vi "PH_uOPA_DelayController.panel.vi"(0 "object ref":refnum<vi>, 5 "error in (no error)":errorcluster) -> (19 "error out":errorcluster)   [LabVIEW 2014, in "PH_uOPA_DelayController.lvlib"]
doc: "This a GUI.\n\nLicense Agreement for this software:\n\nCopyright (C)\nGesellschaft für Schwerionenforschung, GSI\nPlanckstr. 1\n64291 Darmstadt\nGermany\n\nContact: D.Beck@gsi.de \n\nThis program is free software; you can redistribute it and/or modify it under the terms of the GNU General Public License as published by the Free Software Foundation; either version 2 of the license, or (at your option) any later version.\n\nThis program is distributed in the hope that it will be useful, but WITHOUT ANYW ARRANTY; without even the implied warranty of MERCHANTABILITY or FITNESS FOR A PARTICULAR PURPOSE. See the GNU General License for more details (http://www.gnu.org).\n\nGesellschaft für Schwerionenforschung, GSI\nPlanckstr. 1, 64291 Darmstadt, Germany\nFor all questions and ideas contact: M.Richter@gsi.de, H.Brand@gsi.de or D.Beck@gsi.de.\nLast update: 18-DEC-2002"
uses:
  PH_uOPA_DelayController.lvlib
  PH_Basics/PH_StatusHandler/PH_StatusHandler.GUI element.ctl
  PH_Devices/PH_TKTDS-30xx/PH_TKTDS-30xx.Channel Config.ctl
  PH_Devices/PH_TKTDS-30xx/PH_TKTDS-30xx.Waveform Limits.ctl
  PH_Devices/PH_TKTDS-30xx/PH_TKTDS-30xx.Acquisition Config.ctl
  PH_Devices/PH_TKTDS-30xx/PH_TKTDS-30xx.Trigger Config.ctl
  PH_Basics/PH_Stepmotor_BaseClass/PH_Stepmotor_BaseClass.Axis Settings.ctl
  PH_Basics/PH_Stepmotor_BaseClass/PH_Stepmotor_BaseClass.Motor Type.ctl
  PH_Basics/PH_Stepmotor_BaseClass/PH_Stepmotor_BaseClass.Axis Address.ctl
  PH_Basics/PH_Stepmotor_BaseClass/PH_Stepmotor_BaseClass.Axis Activity.ctl
  PH_uOPA_DelayController.Limit.ctl
  PH_uOPA_DelayController.Control Status.ctl
  PH_Devices/PH_TKTDS-30xx/PH_TKTDS-30xx.GUI Refs.ctl
  PH_Basics/PH_AxisGUI_BaseClass/PH_AxisGUI_BaseClass.Axis GUI Refs.ctl
  PH_Basics/PH_Stepmotor_BaseClass/PH_Stepmotor_BaseClass.Axis Direction.ctl
  CS_Core/CSObj/CSObj.lvlib
  PH_Basics/PH_Common/PH_Common.lvlib
  CS_Core/CSSystem/CSSystemLib/CSSystemLib.lvlib
  PH_Devices/PH_TKTDS-30xx/PH_TKTDS-30xx.lvlib
  PH_Basics/PH_Class/PH_Class.lvlib
  PH_Basics/PH_StatusHandler/PH_StatusHandler.lvlib
  PH_Basics/PH_AxisGUI_BaseClass/PH_AxisGUI_BaseClass.lvlib
  PH_Basics/PH_Stepmotor_BaseClass/PH_Stepmotor_BaseClass.lvlib
panel:
  in  "Stop":bool caption="SetZero"
  out "VISA Resource":string
  out "State":u32(colorbox)
  in  "Tab Control":T1(tab)
  out "Current uOPA Mean":dbl caption="uOPA Mean"
  out "Control Status":T2
  in  "Control":bool
  out "Pump running":bool
  in  "Pump Limit [%]":dbl caption="Limit [%]"
  in  "Pump Target":dbl caption="Target"
  in  "uOPA Target":dbl caption="Target"
  in  "uOPA Limits [%]":T3 caption="Limits [%]"
  out "Current uOPA Peak":dbl caption="uOPA Peak"
  out "Current Pump Peak":dbl caption="Pump Peak" format="%_4f"
  out "Activity":T4
  out "Motion Status Bar":u32(colorbox)=16777088 caption="Axis1"
  out "Motion Status":u32(colorbox)=6618880 caption="Axis1"
  in  "Clear Error":bool
  in  "Forth":bool caption="? Steps"
  in  "Back":bool caption="? Steps"
  in  "Target":string="0" caption="Steps"
  out "Trace Pump":waveform(dbl)[](graph)
  out "Trace uOPA":waveform(dbl)[](graph)
  in  "Samples":i32=100
  out "uOPA Mean":dbl(graph)
  out "Pump Peak":dbl(graph)
  out "uOPA Peak":dbl(graph)
  out "Address":T5={"Instance"="N/A", "Motor Nr"=0}
  in  "SetZero":bool
  in  "Reset":bool
  in  "Settings":T6={"Sign change"=FALSE, "Width"=0.0, "Calibration"=0.0, "Unit"="Steps", "Motor Type"=enum."Unspecific", "Unit Width"="", "Unit CF"=""}
  in  "Trigger":T8={"Source"="CH1", "Slope"=0, "Level [V]"=0.0} {"Level [V]" format="%#_6p"}
  in  "Acquisition":T9={"Time base"=2e-07, "Record Length"=10000, "Start Time"=0.0, "Type"=0, "Continuous"=FALSE} {"Start Time" format="%#_12p"; "Record Length" items=["500"=500, "10000"=10000]; "Time base" items=["2ns"=2e-09, "4ns"=4e-09, "10ns"=1e-08, "20ns"=2e-08, "40ns"=4e-08, "100ns"=1e-07, "200ns"=2e-07, "400ns"=4e-07, "1µs"=1e-06, "2µs"=2e-06, "4µs"=4e-06, "10µs"=1e-05, "20µs"=2e-05, "40µs"=4e-05, "100µs"=0.0001, "200µs"=0.0002, "400µs"=0.0004, "1ms"=0.001, "2ms"=0.002, "10ms"=0.01, "20ms"=0.02, "40ms"=0.04, "100ms"=0.1, "200ms"=0.2, "400ms"=0.4, "1s"=1.0, "2s"=2.0, "4s"=4.0, "10s"=10.0]}
  in  "Pump":T10={"Channel Name"="CH1", "Input Impedance"="MEG", "Max Input Frequency"="TWENTY", "Vertical Coupling"=1, "Channel Enabled"=TRUE, "Probe Attenuation"=1.0, "Vertical Range"=100.0, "Vertical Offset"=0.0, "Waveform Limits"={"Start"=1, "End"=10000}} {"Vertical Offset" format="%#_6p"; "Vertical Range" items=["1mV"=0.001, "2mV"=0.002, "5mV"=0.005, "10mV"=0.01, "20mV"=0.02, "50mV"=0.05, "100mV"=0.1, "200mV"=0.2, "500mV"=0.5, "1V"=1.0]; "Probe Attenuation" format="%#.2f"}
  in  "uOPA":T10={"Channel Name"="CH1", "Input Impedance"="MEG", "Max Input Frequency"="TWENTY", "Vertical Coupling"=1, "Channel Enabled"=TRUE, "Probe Attenuation"=1.0, "Vertical Range"=100.0, "Vertical Offset"=0.0, "Waveform Limits"={"Start"=1, "End"=10000}} {"Vertical Offset" format="%#_6p"; "Vertical Range" items=["1mV"=0.001, "2mV"=0.002, "5mV"=0.005, "10mV"=0.01, "20mV"=0.02, "50mV"=0.05, "100mV"=0.1, "200mV"=0.2, "500mV"=0.5, "1V"=1.0]; "Probe Attenuation" format="%#.2f"}
  in  "Position":dbl
  in  "Channel to be positioned":string(combo)="CH1"
  in  "Display Intensity":u8=1 min=1 max=100 step=1
  out "PSDB Status":u32(colorbox)=6618880 caption="PSDB"
  out "Status":T12 caption="Enabling State"
  in  "Delete":bool
  in  "Exit":bool
  # "PCS"
  # "3.40"
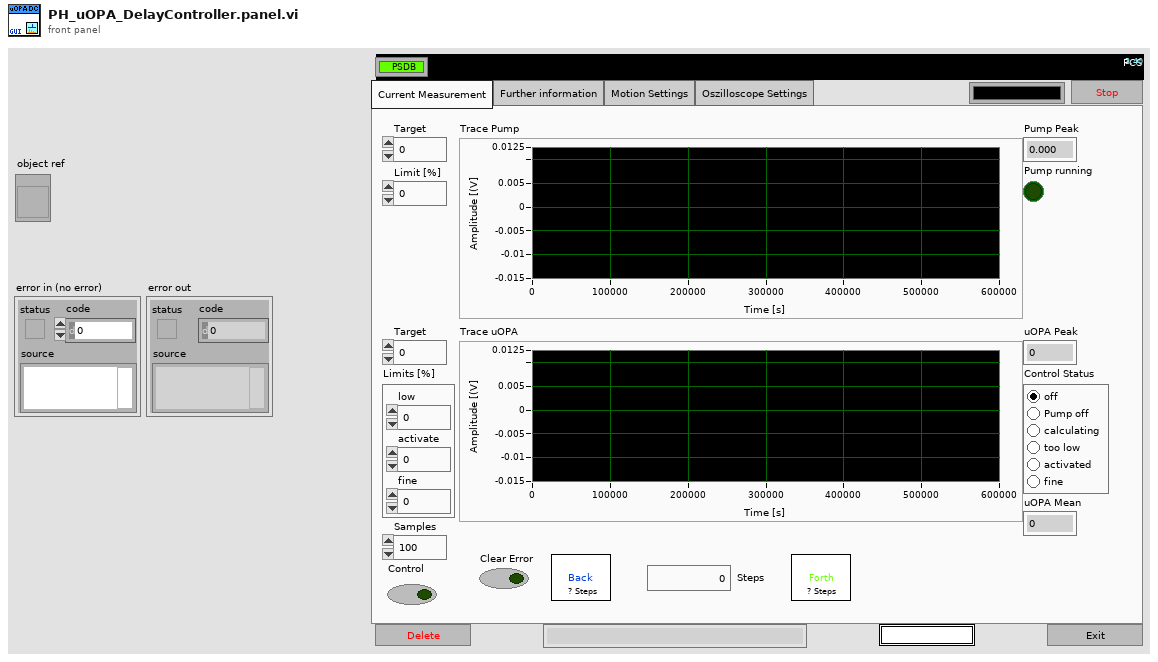
[diagram p1: front panel]
types:
  T1 = enum32{"Current Measurement", "Further information", "Motion Settings", "Oszilloscope Settings"}
  T2 = typedef "PH_uOPA_DelayController.lvlib/PH_uOPA_DelayController.Control Status.ctl" = enum32{"off", "Pump off", "calculating", "too low", "activated", "fine"}
  T3 = typedef "PH_uOPA_DelayController.lvlib/PH_uOPA_DelayController.Limit.ctl" = cluster{"low":dbl, "activate":dbl, "fine":dbl}
  T4 = typedef "PH_Stepmotor_BaseClass.lvlib/PH_Stepmotor_BaseClass.Axis Activity.ctl" = enum16{"No Information", "stopped", "running", "Failure", "Alarm", "stopped at backward ES", "stopped at foreward ES"}
  T5 = typedef "PH_Stepmotor_BaseClass.lvlib/PH_Stepmotor_BaseClass.Axis Address.ctl" = cluster{"Instance":string, "Motor Nr":i32}
  T6 = typedef "PH_Stepmotor_BaseClass.lvlib/PH_Stepmotor_BaseClass.Axis Settings.ctl" = cluster{"Sign change":bool, "Width":dbl, "Calibration":dbl, "Unit":string, "Motor Type":T7, "Unit Width":string, "Unit CF":string}
  T7 = typedef "PH_Stepmotor_BaseClass.lvlib/PH_Stepmotor_BaseClass.Motor Type.ctl" = enum16{"Unspecific", "OWIS 49.120.2633", "OWIS 49.060.1033", "OWIS 43.040.2558", "Diamond Motion 2200 series", "OWIS 49.120.266B.MV6", "Calorimeter", "Linear Stage 1", "MICOS VT-80", "MICOS VT-80 S", "Standa Rotstage nt0.95A", "PUF RA 320.200", "PUF RA 800.200", "PUF RA 800.400", "PUF RA 400.50", "1324.nn.800.50", "1324.n9c.800.50", "1324.nn.320.200", "1324.nn.400.200", "1324.nn.800.200", "1324.nn.400.50", "1324.8c9c.800.50", "1324.8c9c.400.200"}
  T8 = typedef "PH_TKTDS-30xx.lvlib/PH_TKTDS-30xx.Trigger Config.ctl" = cluster{"Source":string, "Slope":i32, "Level [V]":dbl}
  T9 = typedef "PH_TKTDS-30xx.lvlib/PH_TKTDS-30xx.Acquisition Config.ctl" = cluster{"Time base":dbl, "Record Length":u16, "Start Time":dbl, "Type":i32, "Continuous":bool}
  T10 = typedef "PH_TKTDS-30xx.lvlib/PH_TKTDS-30xx.Channel Config.ctl" = cluster{"Channel Name":string, "Input Impedance":string, "Max Input Frequency":string, "Vertical Coupling":i32, "Channel Enabled":bool, "Probe Attenuation":dbl, "Vertical Range":dbl, "Vertical Offset":dbl, "Waveform Limits":T11}
  T11 = typedef "PH_TKTDS-30xx.lvlib/PH_TKTDS-30xx.Waveform Limits.ctl" = cluster{"Start":i32, "End":i32}
  T12 = typedef "PH_StatusHandler.lvlib/PH_StatusHandler.GUI element.ctl" = u16
  T13 = typedef "PH_AxisGUI_BaseClass.lvlib/PH_AxisGUI_BaseClass.Axis GUI Refs.ctl" = cluster{"Back":refnum<vi>, "Forth":refnum<vi>, "Status":refnum<vi>, "Target":refnum<vi>, "Address":refnum<vi>, "Status Bar":refnum<vi>, "Settings":refnum<vi>, "Activity":refnum<vi>, "Clear Error":refnum<vi>}
  T14 = typedef "PH_TKTDS-30xx.lvlib/PH_TKTDS-30xx.GUI Refs.ctl" = cluster{"Trigger":refnum<vi>, "Acquisition":refnum<vi>, "State":refnum<vi>, "Delete":refnum<vi>, "Channel to be positioned":refnum<vi>, "Postion":refnum<vi>, "Display Intensity":refnum<vi>, "VISA Resource":refnum<vi>, "Channels":refnum<vi>[], "Graphs":refnum<vi>[]}
  T15 = typedef "PH_Stepmotor_BaseClass.lvlib/PH_Stepmotor_BaseClass.Axis Direction.ctl" = enum16{"forward", "backward"}
  T16 = typedef "PH_AxisGUI_BaseClass.lvlib/PH_AxisGUI_BaseClass.i attribute.ctl" = cluster{"Axes":T17[]}
  T17 = typedef "PH_AxisGUI_BaseClass.lvlib/PH_AxisGUI_BaseClass.Axis Attributes.ctl" = cluster{"Axis GUI Refs":T13, "Address":T5, "Name":string, "Label \"Back\"":string, "Labell \"Forth\"":string, "Moving?":bool}
  T18 = typedef "PH_uOPA_DelayController.lvlib/PH_uOPA_DelayController.i attribute.ctl" = cluster{"GUI Refs":cluster{"Current Pump Peak":refnum<vi>, "Current uOPA Peak":refnum<vi>, "Pump Peak":refnum<vi>, "uOPA Peak":refnum<vi>, "uOPA Target":refnum<vi>, "uOPA Limits [%]":refnum<vi>, "sample length":refnum<vi>, "Pump Target":refnum<vi>, "Pump Limit":refnum<vi>, "Pump running":refnum<vi>, "Feedback Control":refnum<vi>, "Control Status":refnum<vi>, "uOPA Mean":refnum<vi>, "Current uOPA Mean":refnum<vi>}, "uOPA Target":dbl, "uOPA Limits [%]":T3, "Sample Length":i32, "Initialize Mean":bool, "Pump Target":dbl, "Pump Limit [%]":dbl, "Feedback Control":bool, "Control Status":T2, "last Mean":dbl, "last direction":T15, "Axis Settings":T6, "Width while feedback":dbl}
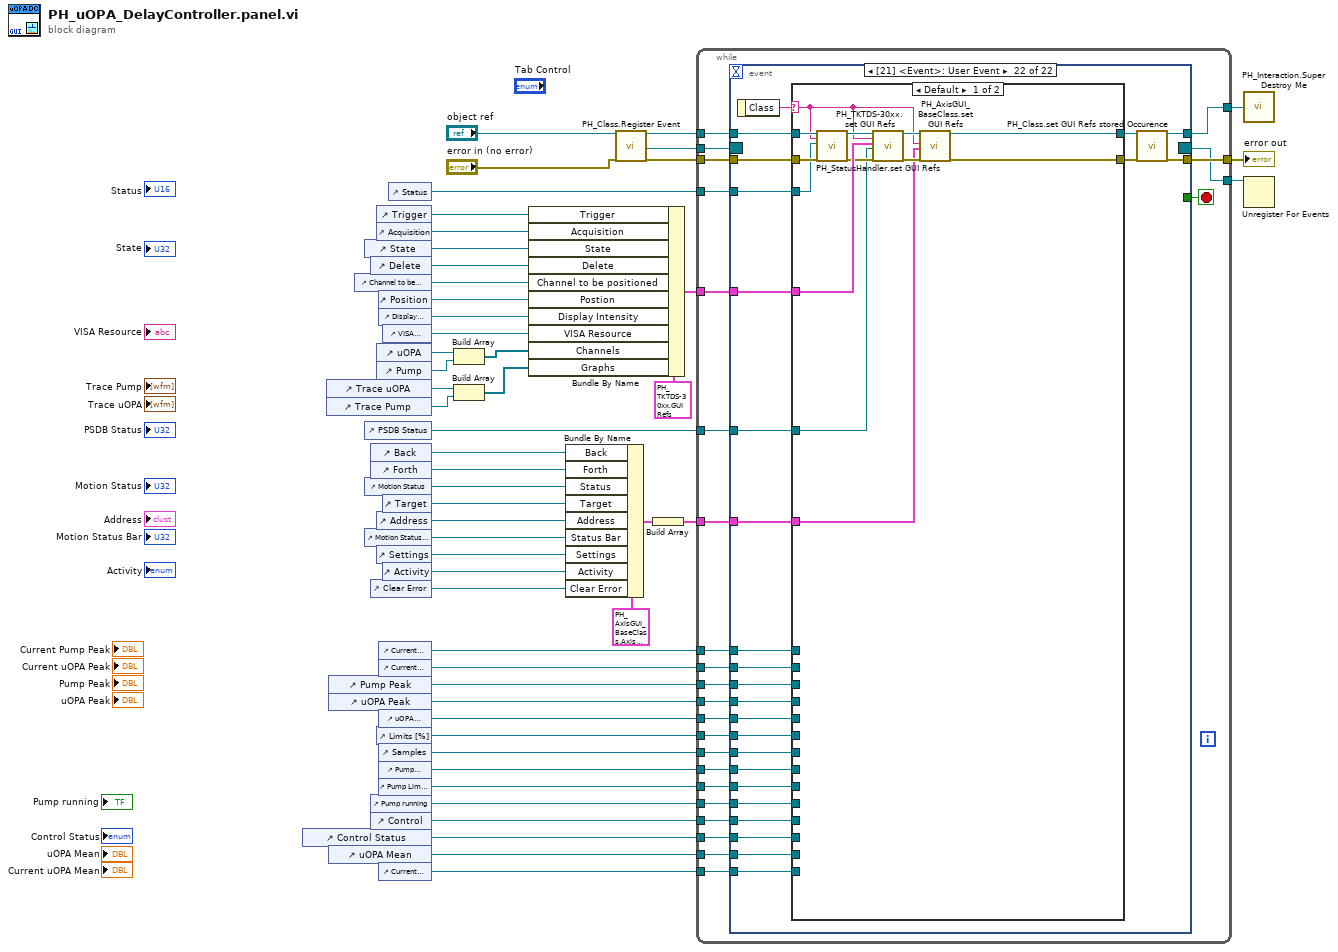
[diagram p0: block diagram]
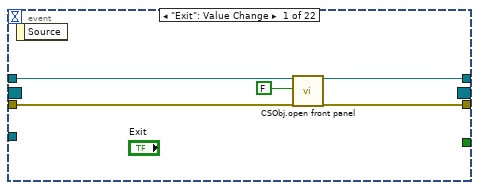
[diagram p2: hidden frame]
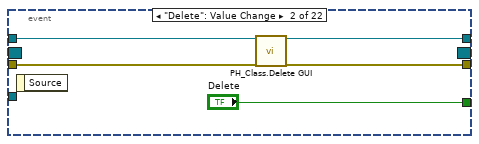
[diagram p3: hidden frame]
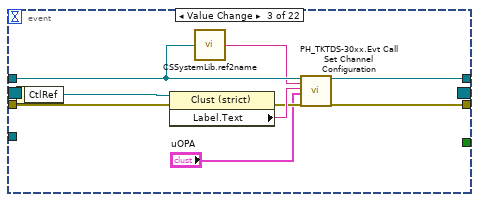
[diagram p4: hidden frame]
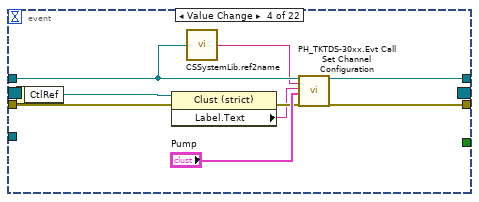
[diagram p5: hidden frame]
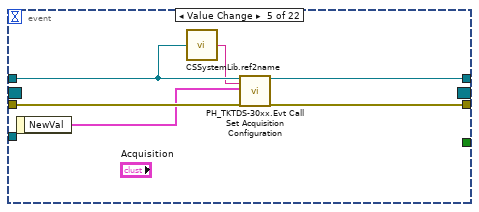
[diagram p6: hidden frame]
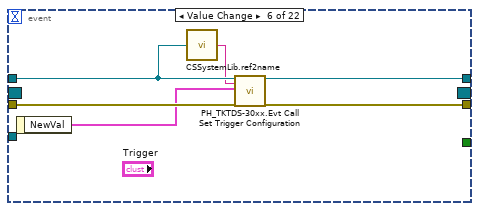
[diagram p7: hidden frame]
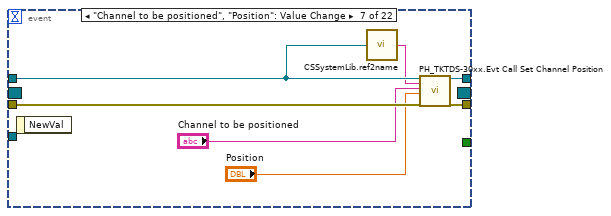
[diagram p8: hidden frame]
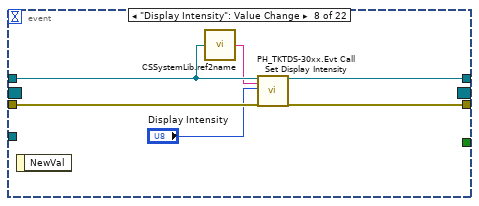
[diagram p9: hidden frame]
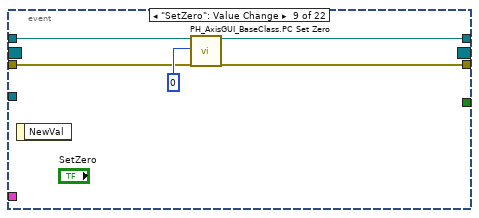
[diagram p10: hidden frame]
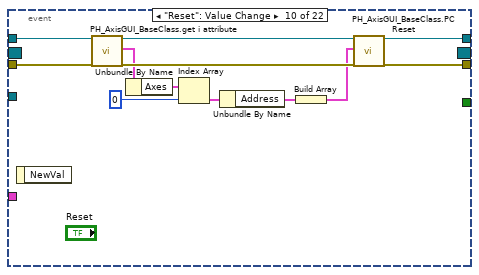
[diagram p11: hidden frame]
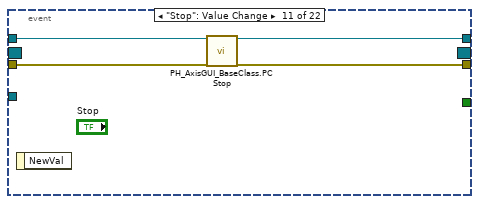
[diagram p12: hidden frame]
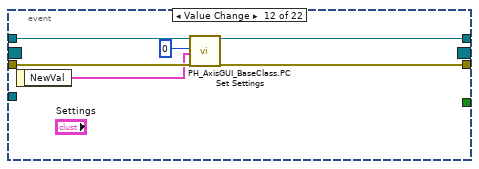
[diagram p13: hidden frame]
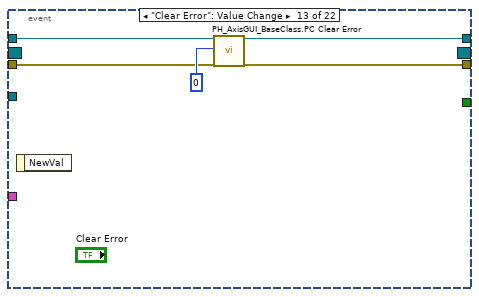
[diagram p14: hidden frame]
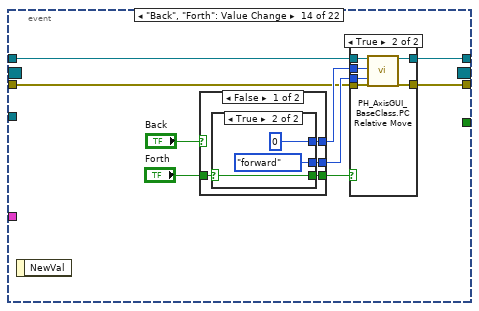
[diagram p15: hidden frame]
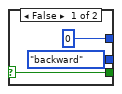
[diagram p16: hidden frame]
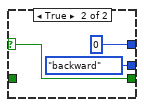
[diagram p17: hidden frame]
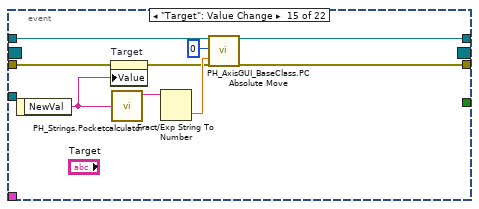
[diagram p19: hidden frame]
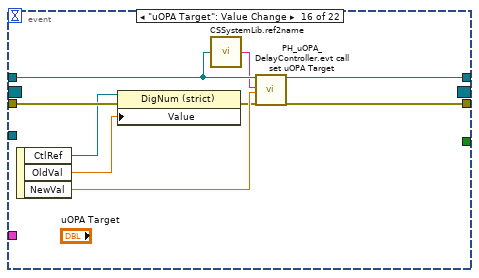
[diagram p20: hidden frame]
diagram:
  n1 = control-ref of="Control Status"() -> (w3:refnum<vi>)
  n2 = control-ref of="Trace uOPA"() -> (w17:refnum<vi>)
  n3 = control-ref of="Trace Pump"() -> (w16:refnum<vi>)
  n4 = control-ref of="Pump Peak"() -> (w12:refnum<vi>)
  n5 = control-ref of="uOPA Peak"() -> (w11:refnum<vi>)
  n6 = control-ref of="uOPA Mean"() -> (w2:refnum<vi>)
  n7 = control-ref of="Channel to be positioned"() -> (w43:refnum<vi>)
  n8 = control-ref of="State"() -> (w45:refnum<vi>)
  n9 = control-ref of="PSDB Status"() -> (w18:refnum<vi>)
  n10 = control-ref of="Motion Status"() -> (w26:refnum<vi>)
  n11 = control-ref of="Motion Status Bar"() -> (w27:refnum<vi>)
  n12 = control-ref of="Delete"() -> (w48:refnum<vi>)
  n13 = control-ref of="Back"() -> (w21:refnum<vi>)
  n14 = control-ref of="Forth"() -> (w20:refnum<vi>)
  n15 = control-ref of="Clear Error"() -> (w19:refnum<vi>)
  n16 = control-ref of="Pump running"() -> (w5:refnum<vi>)
  n17 = control-ref of="Control"() -> (w4:refnum<vi>)
  n18 = control-ref of="Trigger"() -> (w47:refnum<vi>)
  n19 = control-ref of="Acquisition"() -> (w46:refnum<vi>)
  n20 = control-ref of="uOPA"() -> (w50:refnum<vi>)
  n21 = control-ref of="Pump"() -> (w49:refnum<vi>)
  n22 = control-ref of="Address"() -> (w24:refnum<vi>)
  n23 = control-ref of="Settings"() -> (w23:refnum<vi>)
  n24 = control-ref of="Limits [%]"() -> (w9:refnum<vi>)
  n25 = control-ref of="Position"() -> (w42:refnum<vi>)
  n26 = control-ref of="Display Intensity"() -> (w44:refnum<vi>)
  n27 = control-ref of="Current Pump Peak"() -> (w14:refnum<vi>)
  n28 = control-ref of="Current uOPA Peak"() -> (w13:refnum<vi>)
  n29 = control-ref of="uOPA Target"() -> (w10:refnum<vi>)
  n30 = control-ref of="Samples"() -> (w8:refnum<vi>)
  n31 = control-ref of="Pump Target"() -> (w7:refnum<vi>)
  n32 = control-ref of="Pump Limit [%]"() -> (w6:refnum<vi>)
  n33 = control-ref of="Current uOPA Mean"() -> (w1:refnum<vi>)
  n34 = control-ref of="VISA Resource"() -> (w41:refnum<vi>)
  n35 = control-ref of="Target"() -> (w22:refnum<vi>)
  n36 = control-ref of="Activity"() -> (w25:refnum<vi>)
  n37 = control-ref of="Status"() -> (w31:refnum<vi>)
  n38 = Build Array(w50, w49) -> (w35:refnum<vi>[])
  n39 = Build Array(w17, w16) -> (w15:refnum<vi>[])
  n40 = Bundle By Name(cluster=T14 {"Trigger"=refnum, "Acquisition"=refnum, "State"=refnum, "Delete"=refnum, "Channel to be positioned"=refnum, "Postion"=refnum, "Display Intensity"=refnum, "VISA Resource"=refnum, "Channels"=[], "Graphs"=[]} ("GUI Refs"), "Trigger"=w47, "Acquisition"=w46, "State"=w45, "Delete"=w48, "Channel to be positioned"=w43, "Postion"=w42, "Display Intensity"=w44, "VISA Resource"=w41, "Channels"=w35, "Graphs"=w15) -> (w34:T14)
  n41 = Bundle By Name(cluster=T13 {"Back"=refnum, "Forth"=refnum, "Status"=refnum, "Target"=refnum, "Address"=refnum, "Status Bar"=refnum, "Settings"=refnum, "Activity"=refnum, "Clear Error"=refnum} ("GUI Refs"), "Back"=w21, "Forth"=w20, "Status"=w26, "Target"=w22, "Address"=w24, "Status Bar"=w27, "Settings"=w23, "Activity"=w25, "Clear Error"=w19) -> (w29:T13)
  n42 = call "PH_Class.Register Event.vi"("i ref in"="object ref", "error in (no error)"="error in (no error)") -> ("i ref out"=w40:refnum<vi>, "Event Registration Refnum"=w38:refnum<event-registration>, "error out"=w39:errorcluster)  [unwired: 15 in]
  n43 = Build Array(w29) -> (w28:T13[])
  n44 = while {
    tunnel: w40 -> [w74]
    tunnel: [w73] -> w52
    tunnel: w39 -> [w76]
    tunnel: [w75] -> w51
    tunnel: w38 -> [w72]
    tunnel: [w71] -> w37
    tunnel: w31 -> [w70]
    tunnel: w34 -> [w69]
    tunnel: w28 -> [w68]
    tunnel: w18 -> [w67]
    tunnel: w14 -> [w66]
    tunnel: w13 -> [w65]
    tunnel: w12 -> [w64]
    tunnel: w11 -> [w63]
    tunnel: w10 -> [w62]
    tunnel: w9 -> [w61]
    tunnel: w8 -> [w60]
    tunnel: w7 -> [w59]
    tunnel: w6 -> [w58]
    tunnel: w5 -> [w57]
    tunnel: w4 -> [w56]
    tunnel: w3 -> [w55]
    tunnel: w2 -> [w54]
    tunnel: w1 -> [w53]
    stop <- w77 stop-if-true
    n45 = event shown="[21] <Event>: User Event" {
      selector: w72 -> [_ _ _ _ _ _ _ _ _ _ _ _ _ _ _ _ _ _ _ _ _ _]
      dyn-events: [_ _ _ _ _ _ _ _ _ _ _ _ _ _ _ _ _ _ _ _ _ _] -> w71
      timeout: _ -> [_ _ _ _ _ _ _ _ _ _ _ _ _ _ _ _ _ _ _ _ _ _]
      tunnel: [_ "Delete" _ _ _ _ _ _ _ _ _ _ _ _ _ _ _ _ _ _ _ _] -> w77
      tunnel: w74 -> [w79 w84 w94 w103 w108 w114 w121 w127 w134 w139 w151 w156 w161 w168 w198 w207 w216 w225 w234 w243 w252 w278]
      tunnel: w76 -> [w82 w86 w90 w98 w111 w117 w124 w130 w133 w137 w150 w154 w160 w166 w197 w210 w219 w228 w237 w246 w255 w277]
      tunnel: [w81 w85 w96 w105 w110 w116 w123 w129 w131 w136 w148 w153 w158 w165 w194 w208 w217 w226 w235 w244 w253 w279] -> w75
      tunnel: [w78 w83 w95 w104 w109 w115 w122 w128 w132 w138 w149 w155 w159 w167 w195 w209 w218 w227 w236 w245 w254 w280] -> w73
      tunnel: w70 -> [_ _ _ _ _ _ _ _ _ _ _ _ _ _ _ _ _ _ _ _ _ w274]
      tunnel: w69 -> [_ _ _ _ _ _ _ _ _ _ _ _ _ _ _ _ _ _ _ _ _ w272]
      tunnel: w68 -> [_ _ _ _ _ _ _ _ _ _ _ _ _ _ _ _ _ _ _ _ _ w271]
      tunnel: w67 -> [_ _ _ _ _ _ _ _ _ _ _ _ _ _ _ _ _ _ _ _ _ w270]
      tunnel: w66 -> [_ _ _ _ _ _ _ _ _ _ _ _ _ _ _ _ _ _ _ _ _ w269]
      tunnel: w65 -> [_ _ _ _ _ _ _ _ _ _ _ _ _ _ _ _ _ _ _ _ _ w268]
      tunnel: w64 -> [_ _ _ _ _ _ _ _ _ _ _ _ _ _ _ _ _ _ _ _ _ w267]
      tunnel: w63 -> [_ _ _ _ _ _ _ _ _ _ _ _ _ _ _ _ _ _ _ _ _ w266]
      tunnel: w62 -> [_ _ _ _ _ _ _ _ _ _ _ _ _ _ _ _ _ _ _ _ _ w265]
      tunnel: w61 -> [_ _ _ _ _ _ _ _ _ _ _ _ _ _ _ _ _ _ _ _ _ w264]
      tunnel: w60 -> [_ _ _ _ _ _ _ _ _ _ _ _ _ _ _ _ _ _ _ _ _ w263]
      tunnel: w59 -> [_ _ _ _ _ _ _ _ _ _ _ _ _ _ _ _ _ _ _ _ _ w262]
      tunnel: w58 -> [_ _ _ _ _ _ _ _ _ _ _ _ _ _ _ _ _ _ _ _ _ w261]
      tunnel: w57 -> [_ _ _ _ _ _ _ _ _ _ _ _ _ _ _ _ _ _ _ _ _ w260]
      tunnel: w56 -> [_ _ _ _ _ _ _ _ _ _ _ _ _ _ _ _ _ _ _ _ _ w259]
      tunnel: w55 -> [_ _ _ _ _ _ _ _ _ _ _ _ _ _ _ _ _ _ _ _ _ w258]
      tunnel: w54 -> [_ _ _ _ _ _ _ _ _ _ _ _ _ _ _ _ _ _ _ _ _ w257]
      tunnel: w53 -> [_ _ _ _ _ _ _ _ _ _ _ _ _ _ _ _ _ _ _ _ _ w256]
      event "Exit": Value Change {
        n46 = event-data() -> ()  [unwired: 1 in, 1 out]
        n47 = call "CSObj.open front panel.vi"("i ref in"=w79, "frontPanelOpen"=FALSE ("front panel open"), "error in (no error)"=w82) -> ("i ref out"=w78:refnum<vi>, "error out"=w81:errorcluster)  [unwired: 15 in]
      }
      event "Delete": Value Change {
        n48 = event-data() -> ()  [unwired: 1 in, 1 out]
        n49 = call "PH_Class.Delete GUI.vi"("VI in"=w84, "error in (no error)"=w86) -> ("VI out"=w83:refnum<vi>, "error out"=w85:errorcluster)  [unwired: 16 in]
      }
      event Value Change {
        n50 = event-data() -> ("CtlRef"=w93:refnum<vi>)  [unwired: 1 in]
        n51 = property class="Clust (strict)"(reference=w93, error in=w90) -> (error out=w89:errorcluster, "Label.Text"=w91:string)  [unwired: 1 out]
        n52 = call "CSSystemLib.ref2name.vi"("obj refnum"=w94) -> ("name"=w92:string)
        n53 = call "PH_TKTDS-30xx.Evt Call Set Channel Configuration.vi"("i ref in"=w94, "Instance"=w92, "GUI Element Name"=w91, "Channel Configuration"="uOPA", "error in (no error)"=w89) -> ("i ref out"=w95:refnum<vi>, "error out"=w96:errorcluster)  [unwired: 13 in]
      }
      event Value Change {
        n54 = event-data() -> ("CtlRef"=w100:refnum<vi>)  [unwired: 1 in]
        n55 = property class="Clust (strict)"(reference=w100, error in=w98) -> (error out=w99:errorcluster, "Label.Text"=w97:string)  [unwired: 1 out]
        n56 = call "CSSystemLib.ref2name.vi"("obj refnum"=w103) -> ("name"=w102:string)
        n57 = call "PH_TKTDS-30xx.Evt Call Set Channel Configuration.vi"("i ref in"=w103, "Instance"=w102, "GUI Element Name"=w97, "Channel Configuration"="Pump", "error in (no error)"=w99) -> ("i ref out"=w104:refnum<vi>, "error out"=w105:errorcluster)  [unwired: 13 in]
      }
      event Value Change {
        n58 = event-data() -> ("NewVal"=w106:T9)  [unwired: 1 in]
        n59 = call "CSSystemLib.ref2name.vi"("obj refnum"=w108) -> ("name"=w107:string)
        n60 = call "PH_TKTDS-30xx.Evt Call Set Acquisition Configuration.vi"("i ref in"=w108, "Instance"=w107, "Acquisition Configuration"=w106, "error in (no error)"=w111) -> ("i ref out"=w109:refnum<vi>, "error out"=w110:errorcluster)  [unwired: 14 in]
      }
      event Value Change {
        n61 = event-data() -> ("NewVal"=w112:T8)  [unwired: 1 in]
        n62 = call "CSSystemLib.ref2name.vi"("obj refnum"=w114) -> ("name"=w113:string)
        n63 = call "PH_TKTDS-30xx.Evt Call Set Trigger Configuration.vi"("i ref in"=w114, "Instance"=w113, "Trigger Configuration"=w112, "error in (no error)"=w117) -> ("i ref out"=w115:refnum<vi>, "error out"=w116:errorcluster)  [unwired: 14 in]
      }
      event "Channel to be positioned", "Position": Value Change {
        n64 = event-data() -> ()  [unwired: 1 in, 1 out]
        n65 = call "CSSystemLib.ref2name.vi"("obj refnum"=w121) -> ("name"=w120:string)
        n66 = call "PH_TKTDS-30xx.Evt Call Set Channel Position.vi"("i ref in"=w121, "Instance"=w120, "Channel to be positioned"="Channel to be positioned", "Position"="Position", "error in (no error)"=w124) -> ("i ref out"=w122:refnum<vi>, "error out"=w123:errorcluster)  [unwired: 13 in]
      }
      event "Display Intensity": Value Change {
        n67 = event-data() -> ()  [unwired: 1 in, 1 out]
        n68 = call "CSSystemLib.ref2name.vi"("obj refnum"=w127) -> ("name"=w126:string)
        n69 = call "PH_TKTDS-30xx.Evt Call Set Display Intensity.vi"("i ref in"=w127, "Instance"=w126, "Display Intensity"="Display Intensity", "error in (no error)"=w130) -> ("i ref out"=w128:refnum<vi>, "error out"=w129:errorcluster)  [unwired: 14 in]
      }
      event "SetZero": Value Change {
        n70 = event-data() -> ()  [unwired: 1 in, 1 out]
        n71 = call "PH_AxisGUI_BaseClass.PC Set Zero.vi"("VI in"=w134, "Axis"=0 ("index"), "error in (no error)"=w133) -> ("VI out"=w132:refnum<vi>, "error out"=w131:errorcluster)  [unwired: 15 in]
      }
      event "Reset": Value Change {
        n72 = event-data() -> ()  [unwired: 1 in, 1 out]
        n73 = call "PH_AxisGUI_BaseClass.get i attribute.vi"("i ref in"=w139, "error in (no error)"=w137) -> ("i ref out"=w146:refnum<vi>, "i attribute"=w145:T16, "error out"=w147:errorcluster)  [unwired: 15 in]
        n74 = Unbundle By Name(w145) -> ("Axes"=w144:T17[])
        n75 = Index Array(array=w144, index=0) -> (element=w143:T17)
        n76 = Unbundle By Name(w143) -> ("Address"=w142:T5)
        n77 = Build Array(w142) -> (w141:T5[])
        n78 = call "PH_AxisGUI_BaseClass.PC Reset.vi"("i ref in"=w146, "Addresses"=w141, "error in"=w147) -> ("i ref out"=w138:refnum<vi>, "error out"=w136:errorcluster)  [unwired: 15 in]
      }
      event "Stop": Value Change {
        n79 = event-data() -> ()  [unwired: 1 in, 1 out]
        n80 = call "PH_AxisGUI_BaseClass.PC Stop.vi"("VI in"=w151, "error in (no error)"=w150) -> ("VI out"=w149:refnum<vi>, "error out"=w148:errorcluster)  [unwired: 16 in]
      }
      event Value Change {
        n81 = event-data() -> ("NewVal"=w152:T6)  [unwired: 1 in]
        n82 = call "PH_AxisGUI_BaseClass.PC Set Settings.vi"("VI in"=w156, "Axis"=0 ("index"), "NewVal"=w152, "error in (no error)"=w154) -> ("VI out"=w155:refnum<vi>, "error out"=w153:errorcluster)  [unwired: 14 in]
      }
      event "Clear Error": Value Change {
        n83 = event-data() -> ()  [unwired: 1 in, 1 out]
        n84 = call "PH_AxisGUI_BaseClass.PC Clear Error.vi"("i ref in"=w161, "Axis"=0 ("index"), "error in"=w160) -> ("i ref out"=w159:refnum<vi>, "error out"=w158:errorcluster)  [unwired: 15 in]
      }
      event "Back", "Forth": Value Change {
        n85 = event-data() -> ()  [unwired: 1 in, 1 out]
        n86 = case shown="False" "Back" {
          selector: "Back" -> [_ w182]
          tunnel: [w175 0] -> w170
          tunnel: [w174 PH_Stepmotor_BaseClass.Axis_Direction."backward" ("direction")] -> w171
          tunnel: "Forth" -> [w173 _]
          tunnel: [w172 w182] -> w169
          frame False {
            n87 = case shown="True" w173 {
              selector: w173 -> [w176 w179]
              tunnel: [0 0] -> w175
              tunnel: [PH_Stepmotor_BaseClass.Axis_Direction."backward" ("direction") PH_Stepmotor_BaseClass.Axis_Direction."forward" ("direction")] -> w174
              tunnel: [w176 w179] -> w172
              frame False {
              }
              frame True {
              }
            }
          }
          frame True {
          }
        }
        n88 = case shown="True" w169 {
          tunnel: w166 -> [w185 w192]
          tunnel: w168 -> [w186 w191]
          tunnel: w171 -> [_ w190]
          tunnel: [w186 w189] -> w167
          tunnel: [w185 w188] -> w165
          tunnel: w170 -> [_ w187]
          frame False {
          }
          frame True {
            n89 = call "PH_AxisGUI_BaseClass.PC Relative Move.vi"("i ref in"=w191, "Axis"=w187, "direction"=w190, "error in"=w192) -> ("i ref out"=w189:refnum<vi>, "error out"=w188:errorcluster)  [unwired: 14 in]
          }
        }
      }
      event "Target": Value Change {
        n90 = event-data() -> ("NewVal"=w193:string)  [unwired: 1 in]
        n91 = property on="Target" class="Str"(error in=w197, "Value"=w193) -> (error out=w196:errorcluster)  [unwired: 1 in, 1 out]
        n92 = call "PH_Strings.Pocketcalculator.vi"("Input"=w193) -> ("String Double"=w201:string)  [unwired: 3 out]
        n93 = Fract/Exp String To Number(string=w201) -> (number=w200:dbl)  [unwired: 3 in, 1 out]
        n94 = call "PH_AxisGUI_BaseClass.PC Absolute Move.vi"("i ref in"=w198, "Axis"=0, "Position [Units]"=w200, "error in"=w196) -> ("i ref out"=w195:refnum<vi>, "error out"=w194:errorcluster)  [unwired: 14 in]
      }
      event "uOPA Target": Value Change {
        n95 = event-data() -> ("CtlRef"=w203:refnum<vi>, "OldVal"=w202:dbl, "NewVal"=w205:dbl)  [unwired: 1 in]
        n96 = property class="DigNum (strict)"(reference=w203, error in=w210, "Value"=w202) -> (error out=w204:errorcluster)  [unwired: 1 out]
        n97 = call "CSSystemLib.ref2name.vi"("obj refnum"=w207) -> ("name"=w206:string)
        n98 = call "PH_uOPA_DelayController.evt call set uOPA Target.vi"("i ref in"=w207, "Instance"=w206, "uOPA Target"=w205, "error in (no error)"=w204) -> ("i ref out"=w209:refnum<vi>, "error out"=w208:errorcluster)  [unwired: 14 in]
      }
      event "Pump Target": Value Change {
        n99 = event-data() -> ("CtlRef"=w212:refnum<vi>, "OldVal"=w211:dbl, "NewVal"=w214:dbl)  [unwired: 1 in]
        n100 = property class="DigNum (strict)"(reference=w212, error in=w219, "Value"=w211) -> (error out=w213:errorcluster)  [unwired: 1 out]
        n101 = call "CSSystemLib.ref2name.vi"("obj refnum"=w216) -> ("name"=w215:string)
        n102 = call "PH_uOPA_DelayController.evt call set Pump Target.vi"("i ref in"=w216, "Instance"=w215, "Pump Target"=w214, "error in (no error)"=w213) -> ("i ref out"=w218:refnum<vi>, "error out"=w217:errorcluster)  [unwired: 14 in]
      }
      event "Pump Limit [%]": Value Change {
        n103 = event-data() -> ("CtlRef"=w221:refnum<vi>, "OldVal"=w220:dbl, "NewVal"=w223:dbl)  [unwired: 1 in]
        n104 = property class="DigNum (strict)"(reference=w221, error in=w228, "Value"=w220) -> (error out=w222:errorcluster)  [unwired: 1 out]
        n105 = call "CSSystemLib.ref2name.vi"("obj refnum"=w225) -> ("name"=w224:string)
        n106 = call "PH_uOPA_DelayController.evt call set Pump Limit.vi"("i ref in"=w225, "Instance"=w224, "Pump Limit"=w223, "error in (no error)"=w222) -> ("i ref out"=w227:refnum<vi>, "error out"=w226:errorcluster)  [unwired: 14 in]
      }
      event Value Change {
        n107 = event-data() -> ("CtlRef"=w230:refnum<vi>, "OldVal"=w229:T3, "NewVal"=w232:T3)  [unwired: 1 in]
        n108 = property class="Clust (strict)"(reference=w230, error in=w237, "Value"=w229) -> (error out=w231:errorcluster)  [unwired: 1 out]
        n109 = call "CSSystemLib.ref2name.vi"("obj refnum"=w234) -> ("name"=w233:string)
        n110 = call "PH_uOPA_DelayController.evt call set uOPA Limits.vi"("i ref in"=w234, "Instance"=w233, "Limits [%]"=w232, "error in (no error)"=w231) -> ("i ref out"=w236:refnum<vi>, "error out"=w235:errorcluster)  [unwired: 14 in]
      }
      event "Samples": Value Change {
        n111 = event-data() -> ("CtlRef"=w240:refnum<vi>, "OldVal"=w239:i32, "NewVal"=w238:i32)  [unwired: 1 in]
        n112 = property class="DigNum (strict)"(reference=w240, error in=w246, "Value"=w239) -> (error out=w241:errorcluster)  [unwired: 1 out]
        n113 = call "CSSystemLib.ref2name.vi"("obj refnum"=w243) -> ("name"=w242:string)
        n114 = call "PH_uOPA_DelayController.evt call set Sample Length.vi"("i ref in"=w243, "Instance"=w242, "Sample Length"=w238, "error in (no error)"=w241) -> ("i ref out"=w245:refnum<vi>, "error out"=w244:errorcluster)  [unwired: 14 in]
      }
      event "Control": Value Change {
        n115 = event-data() -> ("CtlRef"=w249:refnum<vi>, "OldVal"=w248:bool, "NewVal"=w247:bool)  [unwired: 1 in]
        n116 = property class="Bool (strict)"(reference=w249, error in=w255, "Value"=w248) -> (error out=w250:errorcluster)  [unwired: 1 out]
        n117 = call "CSSystemLib.ref2name.vi"("obj refnum"=w252) -> ("name"=w251:string)
        n118 = call "PH_uOPA_DelayController.evt call set Feedback Control.vi"("i ref in"=w252, "Instance"=w251, "Feedback Control"=w247, "error in (no error)"=w250) -> ("i ref out"=w254:refnum<vi>, "error out"=w253:errorcluster)  [unwired: 14 in]
      }
      event User Event {
        n119 = event-data() -> ("Class"=w273:string)  [unwired: 1 in]
        n120 = case shown="Default" w273 {
          selector: w273 -> [w282 _]
          tunnel: w278 -> [w290 w315]
          tunnel: w277 -> [w293 w314]
          tunnel: [w286 w311] -> w276
          tunnel: [w284 w310] -> w275
          tunnel: w274 -> [w288 _]
          tunnel: w272 -> [w292 _]
          tunnel: w271 -> [w283 _]
          tunnel: w270 -> [w281 _]
          tunnel: w269 -> [_ w307]
          tunnel: w268 -> [_ w306]
          tunnel: w267 -> [_ w305]
          tunnel: w266 -> [_ w304]
          tunnel: w265 -> [_ w303]
          tunnel: w264 -> [_ w302]
          tunnel: w263 -> [_ w301]
          tunnel: w262 -> [_ w300]
          tunnel: w261 -> [_ w299]
          tunnel: w260 -> [_ w298]
          tunnel: w259 -> [_ w297]
          tunnel: w258 -> [_ w296]
          tunnel: w257 -> [_ w295]
          tunnel: w256 -> [_ w294]
          frame Default {
            n121 = call "PH_StatusHandler.set GUI Refs.vi"("i ref in"=w290, "Class"=w282, "GUI Ref"=w288, "error in (no error)"=w293) -> ("i ref out"=w289:refnum<vi>, "error out"=w291:errorcluster)  [unwired: 14 in]
            n122 = call "PH_TKTDS-30xx.set GUI Refs.vi"("i ref in"=w289, "Class"=w282, "GUI Refs"=w292, "Ref PSDB Status"=w281, "error in (no error)"=w291) -> ("i ref out"=w287:refnum<vi>, "error out"=w285:errorcluster)  [unwired: 13 in]
            n123 = call "PH_AxisGUI_BaseClass.set GUI Refs.vi"("i ref in"=w287, "Class"=w282, "Axis GUI Base Class Refs"=w283, "error in"=w285) -> ("i ref out"=w286:refnum<vi>, "error out"=w284:errorcluster)  [unwired: 14 in]
          }
          frame "PH_uOPA_DelayController" {
            n124 = call "PH_uOPA_DelayController.get data to modify.vi"("i ref in"=w315, "ms timeout (10000)"=-1, "error in (no error)"=w314) -> ("i ref out"=w316:refnum<vi>, "i attribute"=w309:T18, "error out"=w317:errorcluster)  [unwired: 13 in, 1 out]
            n125 = Bundle By Name(cluster=w309, "GUI Refs.Current Pump Peak"=w307, "GUI Refs.Current uOPA Peak"=w306, "GUI Refs.Pump Peak"=w305, "GUI Refs.uOPA Peak"=w304, "GUI Refs.uOPA Target"=w303, "GUI Refs.uOPA Limits [%]"=w302, "GUI Refs.sample length"=w301, "GUI Refs.Pump Target"=w300, "GUI Refs.Pump Limit"=w299, "GUI Refs.Pump running"=w298, "GUI Refs.Feedback Control"=w297, "GUI Refs.Control Status"=w296, "GUI Refs.uOPA Mean"=w295, "GUI Refs.Current uOPA Mean"=w294) -> (w308:T18)
            n126 = call "PH_uOPA_DelayController.set modified data.vi"("i ref in"=w316, "i attribute"=w308, "error in (no error)"=w317) -> ("i ref out"=w312:refnum<vi>, "error out"=w313:errorcluster)  [unwired: 15 in]
            n127 = call "PH_uOPA_DelayController.initialize GUI.vi"("i ref in"=w312, "error in (no error)"=w313) -> ("i ref out"=w311:refnum<vi>, "error out"=w310:errorcluster)  [unwired: 16 in]
          }
        }
        n128 = call "PH_Class.set GUI Refs stored Occurence.vi"("i ref in"=w276, "error in (no error)"=w275) -> ("i ref out"=w280:refnum<vi>, "error out"=w279:errorcluster)  [unwired: 16 in]
      }
    }
  }
  "error out" <- w51
  n129 = call "PH_Interaction.Super Destroy Me.vi"("i ref out"=w52) -> ()
  n130 = Unregister For Events(event registration refnum=w37) -> ()  [unwired: 1 in, 1 out]
